vi "Create.vi"(8 "error in (no error)":errorcluster, 10 "Input":string) -> (0 "error out":errorcluster, 2 "Label":string, 3 "Proto":refnum<class "Rule.lvclass">)   [LabVIEW 2021, in "Rule.lvclass"]
uses:
  Rule.lvclass
  Rule.lvclass/Rule.ctl
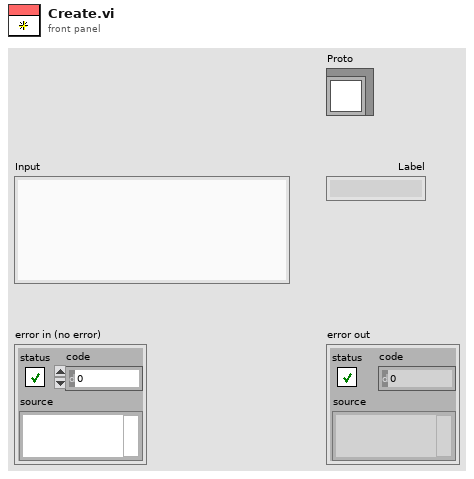
[diagram p1: front panel]
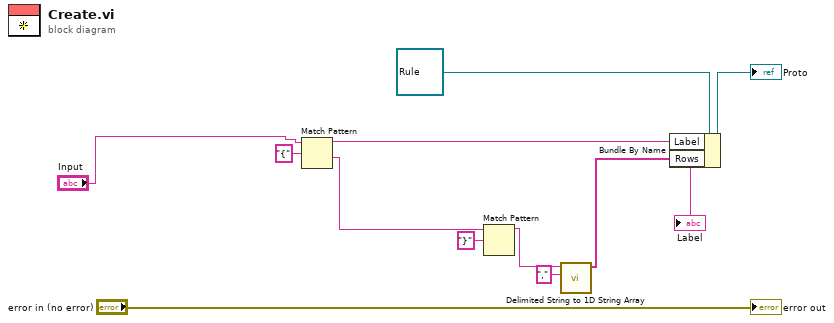
[diagram p0: block diagram]
diagram:
  n1 = Match Pattern(string="Input", regular expression="{") -> (before substring=w6:string, after substring=w5:string)  [unwired: 1 in, 2 out]
  "Label" <- w6
  n2 = Match Pattern(string=w5, regular expression="}") -> (before substring=w3:string)  [unwired: 1 in, 3 out]
  n3 = call <vilib>:"Delimited String to 1D String Array.vi"("delimiter"=",", "delimited string"=w3) -> ("string array"=w1:string[])  [unwired: 9 in]
  n4 = Bundle By Name(cluster=refnum<class "Rule.lvclass"> refnum ("Proto"), "Label"=w6, "Rows"=w1) -> (→"Proto":refnum<class "Rule.lvclass">)
  "error out" <- "error in (no error)"
